vi "Read All.vi"(11 "Collection In":refnum<class "Collection.lvclass">) -> (0 "Coords":T1[](array[typedef]), 3 "Collection Out":refnum<class "Collection.lvclass">)   [LabVIEW 2020, in "Collection.lvclass"]
uses:
  Collection.lvclass
  Coords Cluster.ctl
  Collection.lvclass/Collection.ctl
  Dauntless.lvclass
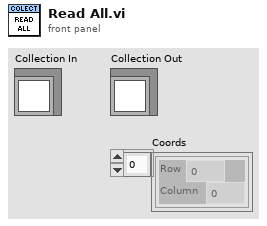
[diagram p1: front panel]
types:
  T1 = typedef "Dauntless.lvclass/Coords Cluster.ctl" = cluster{"Row":i32, "Column":i32}
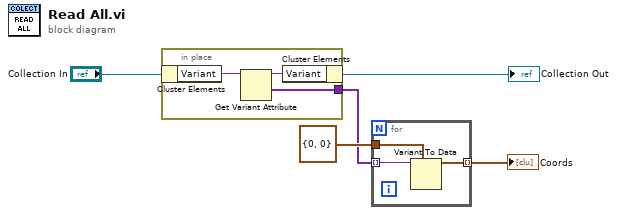
[diagram p0: block diagram]
diagram:
  n1 = in-place {
    in-place-border: [w6] -> w2
    n2 = in-place-cluster #1("Collection In") -> ("Variant"=w8:variant)
    n3 = Get Variant Attribute(Variant=w8) -> (duplicate Variant=w7:variant, values=w6:variant[])  [unwired: 3 in, 2 out]
    n4 = in-place-cluster #1("Variant"=w7) -> (→"Collection Out":refnum<class "Collection.lvclass">)
  }
  n5 = for {
    tunnel: T1 {"Row"=0, "Column"=0} ("Coords") -> [w11]
    tunnel: w2 -> [w10] mode=indexing
    tunnel: [w9] -> w1 mode=indexing
    n6 = Variant To Data(type=w11, Variant=w10) -> (data=w9:T1)  [unwired: 1 in, 1 out]
  }
  "Coords" <- w1
